vi "Do Hall Effect Calculations.vi"(8 "error in (no error)":errorcluster) -> (0 "error out":errorcluster)   [LabVIEW 2016, in "Hall Effect Library.lvlib"]
uses:
  Hall Effect Library.lvlib
  Global Variables/Hall Effect Data.vi
  Global Variables/Test Settings.vi
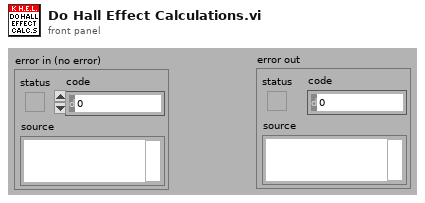
[diagram p1: front panel]
types:
  T1 = cluster{"fA":dbl, "fB":dbl, "QA":dbl, "QB":dbl, "pAvg":dbl, "pA":dbl, "pB":dbl}
  T2 = cluster{"RHD":dbl, "RHC":dbl, "RHAvg":dbl, "uH":dbl, "n/p":dbl}
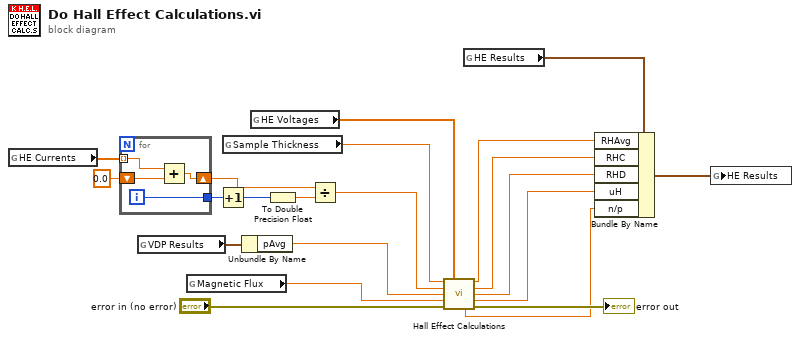
[diagram p0: block diagram]
diagram:
  n1 = global read "Hall Effect Data.vi" "HE Currents"() -> (w17:dbl[])
  n2 = for {
    tunnel: w17 -> [w25] mode=indexing
    shift-right: [w22] -> w11
    shift-left: 0.0 -> [w24]
    tunnel: [w23] -> w3
    i -> [w23]
    n3 = Add(x=w25, y=w24) -> (x+y=w22:dbl)
  }
  n4 = global read "Hall Effect Data.vi" "VDP Results"() -> (w14:T1)
  n5 = global read "Test Settings.vi" "Magnetic Flux"() -> (w12:dbl)
  n6 = Increment(x=w3) -> (x+1=w1:i32)
  n7 = global read "Test Settings.vi" "Sample Thickness"() -> (w18:dbl)
  n8 = Unbundle By Name(w14) -> ("pAvg"=w13:dbl)
  n9 = global read "Hall Effect Data.vi" "HE Voltages"() -> (w19:dbl[])
  n10 = To Double Precision Float(number=w1) -> (double precision float=w2:dbl)
  n11 = Divide(x=w11, y=w2) -> (x/y=w15:dbl)
  n12 = call "Hall Effect Calculations.vi"("Thickness (cm)"=w18, "Hall Voltage Array"=w19, "Current (A)"=w15, "pAVG"=w13, "Flux"=w12, "error"="error in (no error)") -> ("RHAVG"=w9:dbl, "RHC"=w8:dbl, "RHD"=w7:dbl, "Hall Mobility"=w6:dbl, "n/p"=w4:dbl, "error out"=→"error out":errorcluster)  [unwired: 4 out]
  n13 = global read "Hall Effect Data.vi" "HE Results"() -> (w10:T2)
  n14 = Bundle By Name(cluster=w10, "RHAvg"=w9, "RHC"=w8, "RHD"=w7, "uH"=w6, "n/p"=w4) -> (w5:T2)
  n15 = global write "Hall Effect Data.vi" "HE Results"(w5) -> ()
